vi "Lim Inferior.vi"(8 "error in (no error)":errorcluster, 10 "MIN":dbl, 11 "Contador in":refnum<class "Contador.lvclass">) -> (0 "error out":errorcluster, 3 "Contador out":refnum<class "Contador.lvclass">)   [LabVIEW 2020, in "Contador.lvlib" / "Contador.lvclass"]
uses:
  Contador.lvclass
  Contador.lvclass/Contador.ctl
  ACQ Contador/ACQ Contador Messages/Lim Inferior Msg/Lim Inferior Msg.lvclass/Lim Inferior Msg.ctl
  <vilib>/ActorFramework/Message Enqueuer/Message Enqueuer.lvclass/Message Enqueuer.ctl
  <vilib>/ActorFramework/Message Enqueuer/Enqueue.vi
  ACQ Contador/ACQ Contador Messages/Lim Inferior Msg/Lim Inferior Msg.lvclass
  C:/Program Files (x86)/National Instruments/LabVIEW 2020/vi.lib/ActorFramework/Message/Message.lvclass
  <vilib>/ActorFramework/Message Priority Queue/Priority Enqueue.vi
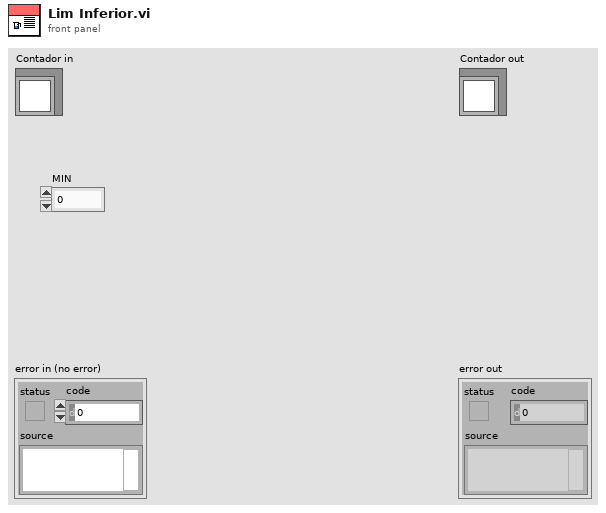
[diagram p1: front panel]
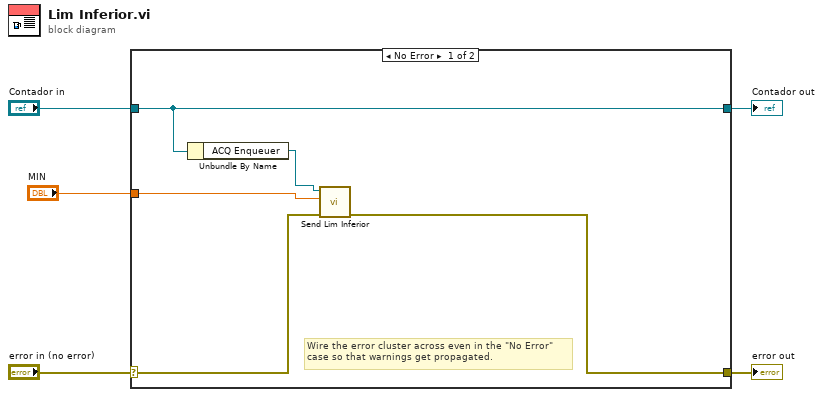
[diagram p0: block diagram]
diagram:
  n1 = case shown="No Error" "error in (no error)" {
    selector: "error in (no error)" -> [w7 w12]
    tunnel: [w6 w12] -> w4
    tunnel: [w10 w11] -> w2
    tunnel: "Contador in" -> [w10 w11]
    tunnel: "MIN" -> [w8 _]
    frame No Error {
      # "Wire the error cluster across even in the \"No Error\"\ncase so that warnings get propagated."
      n2 = Unbundle By Name(w10) -> ("ACQ Enqueuer"=w9:refnum<class "Message Enqueuer.lvclass">)
      n3 = call "Send Lim Inferior.vi"("error in (no error)"=w7, "MIN"=w8, "Message Enqueuer"=w9) -> ("error out"=w6:errorcluster)  [unwired: 7 in, 1 out]
    }
    frame Error {
    }
  }
  "error out" <- w4
  "Contador out" <- w2
